vi "Abort.vi"(8 "error in (no error)":errorcluster, 11 "AcPwrBase in":refnum<class "AcPwrBase.lvclass">) -> (0 "error out":errorcluster, 3 "AcPwrBase out":refnum<class "AcPwrBase.lvclass">)   [LabVIEW 2018, in "AcPwrPlugins.lvlib" / "AcPwrBase.lvclass"]
uses:
  AcPwrBase.lvclass
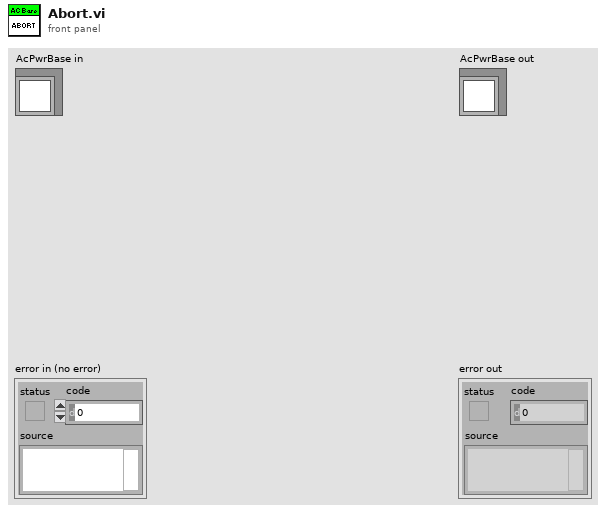
[diagram p1: front panel]
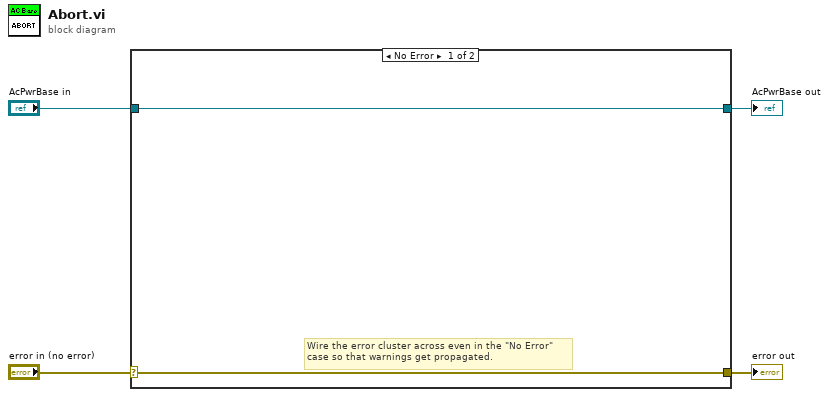
[diagram p0: block diagram]
diagram:
  n1 = case shown="No Error" "error in (no error)" {
    selector: "error in (no error)" -> [w5 w8]
    tunnel: [w5 w8] -> w3
    tunnel: [w6 w7] -> w1
    tunnel: "AcPwrBase in" -> [w6 w7]
    frame No Error {
      # "Wire the error cluster across even in the \"No Error\"\ncase so that warnings get propagated."
    }
    frame Error {
    }
  }
  "error out" <- w3
  "AcPwrBase out" <- w1
